vi "Control Climb.vi"   [LabVIEW 2020]
uses:
  Framework/Robot Global Data.vi
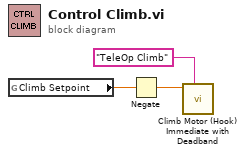
[diagram p0: block diagram]
diagram:
  n1 = global read "Robot Global Data.vi" "Climb Setpoint"() -> (w1:dbl)
  n2 = Negate(x=w1) -> (-x=w2:dbl)
  n3 = call "Climb Motor (Hook) Immediate with Deadband.vi"("Description"="TeleOp Climb", "Setpoint"=w2) -> ()  [unwired: 9 in, 1 out]
